vi "APS absolute move2.vi"(4 "Dec_Rate":i32, 5 "Acc_Rate":i32, 6 "End_Speed":i32, 7 "Max_Speed":i32, 8 "error in (no error)":errorcluster caption="错误输入（无错误）", 9 "Start_Speed":i32, 10 "Position":i32, 11 "Axis_ID":i32) -> (0 "error out":errorcluster caption="错误输出", 3 "function return":i32)   [LabVIEW 2011, in "APS168.lvlib"]
doc: "I32 FNTYPE APS_absolute_move2( I32 Axis_ID, I32 Position, I32 Start_Speed, I32 Max_Speed, I32 End_Speed, I32 Acc_Rate, I32 Dec_Rate );"
uses:
  APS168.lvlib
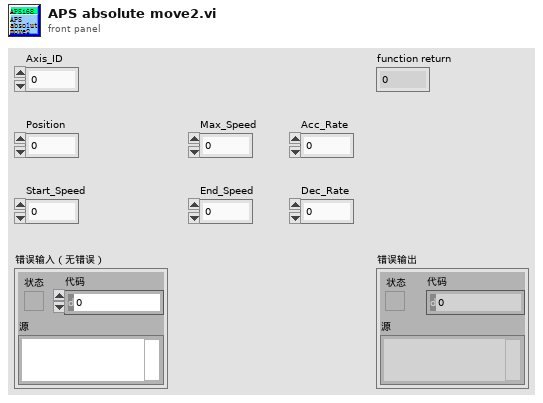
[diagram p1: front panel]
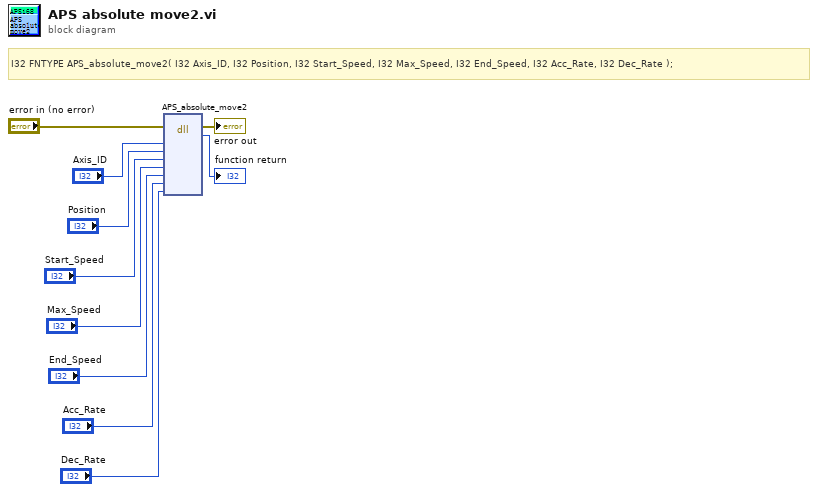
[diagram p0: block diagram]
diagram:
  # "I32 FNTYPE APS_absolute_move2( I32 Axis_ID, I32 Position, I32 Start_Speed, I32 Max_Speed, I32 End_Speed, I32 Acc_Rate, I32 Dec_Rate );"
  n1 = dll-call lib="PTH1Labs E软件ADLINK 204CAPS_1_7_1_LIB line 连续运动204APS168.*" fn="APS_absolute_move2"(error in="error in (no error)", "Axis_ID"="Axis_ID", "Position"="Position", "Start_Speed"="Start_Speed", "Max_Speed"="Max_Speed", "End_Speed"="End_Speed", "Acc_Rate"="Acc_Rate", "Dec_Rate"="Dec_Rate") -> (error out=→"error out":errorcluster, →"function return":i32)  [unwired: 9 in, 1 out]
